vi "PMJD T027 SubVI06.vi"(1 "Q":dbl, 2 "u00":dbl, 3 "upq":dbl, 4 "P":dbl) -> (0 "npq":dbl)   [LabVIEW 2020]
doc: "PINEDA MENDEZ JOB DANIEL 4MV6 SVA 2022/1\nT027 SubVI06 \nCalculo de momentos normalizados npq\nEste subvi obtiene los momentos normalizados a partir de los parametros P,Q, upq, u00"
panel:
  # "PINEDA MENDEZ JOB DANIEL    4MV6    SVA    2022/1\nT027     SubVI06 Calculo de momentos normalizados npq"
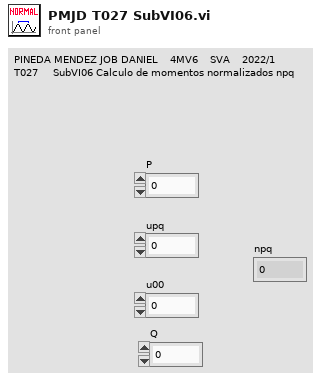
[diagram p1: front panel]
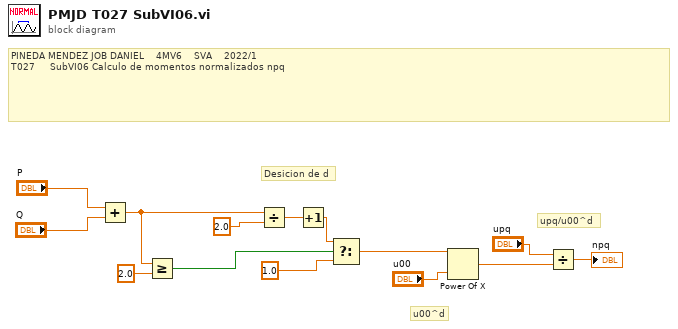
[diagram p0: block diagram]
diagram:
  # "PINEDA MENDEZ JOB DANIEL    4MV6    SVA    2022/1\nT027     SubVI06 Calculo de momentos normalizados npq"
  # "upq/u00^d"
  # "u00^d"
  # "Desicion de d"
  n1 = Add(x="P", y="Q") -> (x+y=w2:dbl)
  n2 = Greater Or Equal?(x=w2, y=2.0) -> (x >= y?=w3:bool)
  n3 = Divide(x=w2, y=2.0) -> (x/y=w6:dbl)
  n4 = Increment(x=w6) -> (x+1=w4:dbl)
  n5 = Select(t=w4, s=w3, f=1.0) -> (s? t:f=w1:dbl)
  n6 = Power Of X(1:"u00", 2:w1) -> (0:w9:dbl)
  n7 = Divide(x="upq", y=w9) -> (x/y=→"npq":dbl)
